vi "Send to Process.vi"(8 "error in (no error)":errorcluster, 9 "message value":variant, 10 "message name":string, 11 "qbus in":refnum<class "Qbus.lvclass">) -> (0 "error out":errorcluster, 3 "qbus out":refnum<class "Qbus.lvclass">)   [LabVIEW 2015, in "Exposure Process.lvlib"]
doc: "Registers an event with the Timer process. When the event timer expires, the timer sends the callback action and value to the specified process."
uses:
  Exposure Process.lvlib
  <vilib>/addons/Qbus/Qbus.lvclass
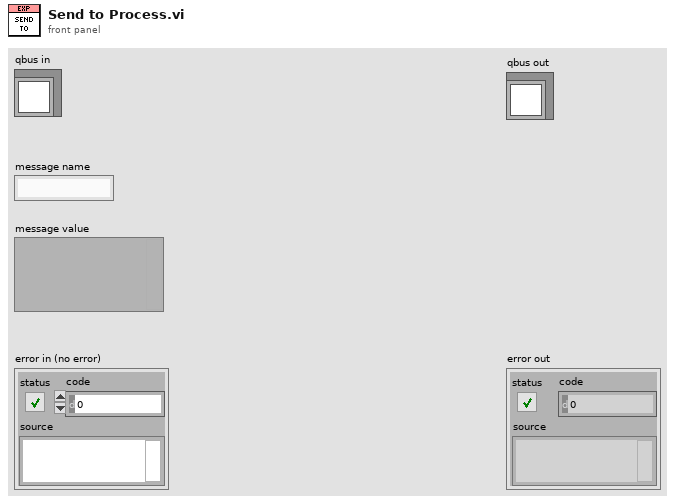
[diagram p1: front panel]
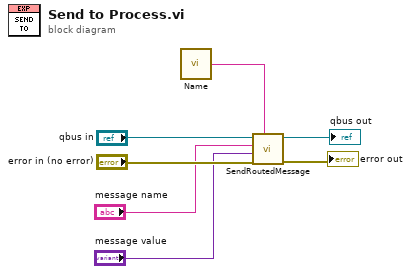
[diagram p0: block diagram]
diagram:
  n1 = call "Name.vi"() -> ("process name"=w6:string)  [unwired: 5 in]
  n2 = call <vilib>:"SendRoutedMessage.vi"("listener process"=w6, "error in (no error)"="error in (no error)", "message value"="message value", "message name"="message name", "Qbus in"="qbus in") -> ("error in (no error)"=→"error out":errorcluster, "Qbus out"=→"qbus out":refnum<class "Qbus.lvclass">)  [unwired: 5 in]
